vi "NIIE_Flip color refs.vi"(6 "Flip colors?":bool, 10 "Shift pressed":bool, 11 "CTRL pressed":bool) -> (3 "Flip?":bool)   [LabVIEW 2021]
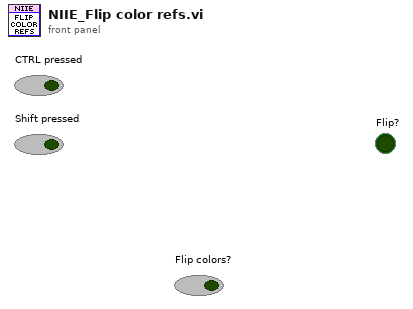
[diagram p1: front panel]
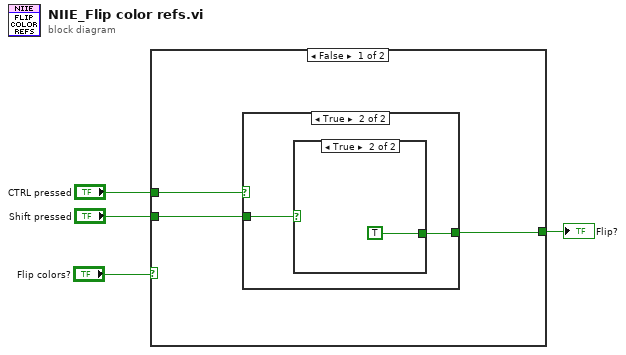
[diagram p0: block diagram]
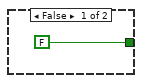
[diagram p2: hidden frame]
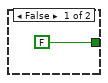
[diagram p3: hidden frame]
diagram:
  n1 = case shown="False" "Flip colors?" {
    selector: "Flip colors?" -> [_ w13]
    tunnel: [w5 w13] -> w3
    tunnel: "CTRL pressed" -> [w7 _]
    tunnel: "Shift pressed" -> [w6 _]
    frame False {
      n2 = case shown="True" w7 {
        tunnel: w6 -> [_ w10]
        tunnel: [FALSE w9] -> w5
        frame False {
        }
        frame True {
          n3 = case shown="True" w10 {
            tunnel: [FALSE TRUE] -> w9
            frame False {
            }
            frame True {
            }
          }
        }
      }
    }
    frame True {
    }
  }
  "Flip?" <- w3
